vi "ApplyIconToLibrary.vi"(8 "error in (no error)":errorcluster, 9 "Apply banner color to class wire":bool=TRUE, 10 "Icon":refnum<class "Icon.lvclass">, 11 "Library Refnum in":refnum<vi>) -> (0 "error out":errorcluster, 3 "Library Refnum out":refnum<vi>)   [LabVIEW 2014, in "BasicClassDocumentation.lvlib" / "BasicClassDocumentation.lvclass"]
uses:
  BasicClassDocumentation.lvclass
  <vilib>/LabVIEW Icon API/lv_icon/Classes/Icon/Icon.lvclass
  <vilib>/LabVIEW Icon API/LabVIEW Icon API.lvlib
  Utilites/_ProjectItemsUtilities/_ProjectItemsUtilities.lvlib
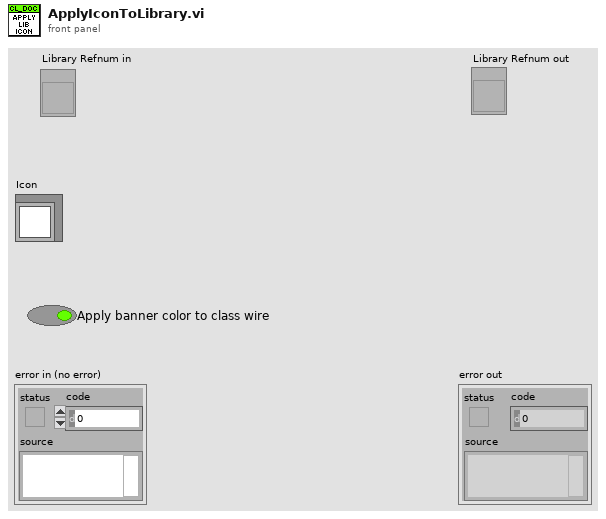
[diagram p1: front panel]
types:
  T1 = typedef "imagedata.ctl" = cluster{"image type":i32, "image depth":i32, "image":u8[], "mask":u8[], "colors":u32[], "Rectangle":cluster{"left":i16, "top":i16, "right":i16, "bottom":i16}}
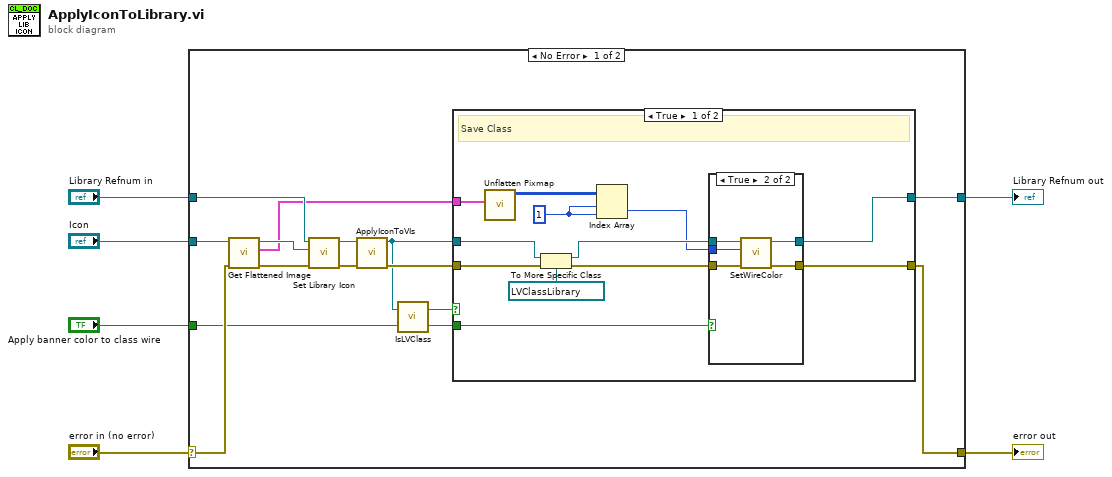
[diagram p0: block diagram]
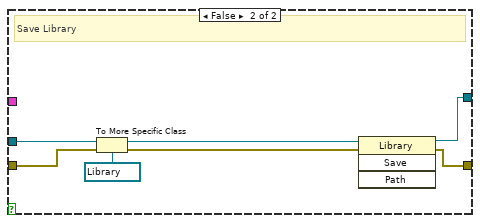
[diagram p3: hidden frame]
diagram:
  n1 = case shown="No Error" "error in (no error)" {
    selector: "error in (no error)" -> [w12 w48]
    tunnel: [w10 w48] -> w5
    tunnel: "Icon" -> [w14 _]
    tunnel: "Library Refnum in" -> [w15 w47]
    tunnel: [w8 w47] -> w2
    tunnel: "Apply banner color to class wire" -> [w7 _]
    frame No Error {
      n2 = call <vilib>:"Get Flattened Image.vi"("error in (no error)"=w12, "lv_icon.lvlib:Icon.lvclass in"=w14) -> ("error out"=w11:errorcluster, "Color Image"=w9:T1, "lv_icon.lvlib:Icon.lvclass out"=w13:refnum<class "Icon.lvclass">)  [unwired: 6 in, 1 out]
      n3 = call <vilib>:"Set Library Icon.vi"("error in (no error)"=w11, "Icon"=w13, "Library Refnum in"=w15) -> ("error out"=w20:errorcluster, "Library Refnum out"=w19:refnum<vi>)  [unwired: 7 in]
      n4 = call "ApplyIconToVIs.vi"("error in (no error)"=w20, "Library Refnum"=w19) -> ("error out"=w18:errorcluster, "Library Refnum out"=w17:refnum<vi>)  [unwired: 8 in]
      n5 = call "IsLVClass.vi"("ProjectItem Refnum"=w17) -> ("IsLVClass?"=w16:bool)  [unwired: 2 in]
      n6 = case shown="True" w16 {
        tunnel: w18 -> [w32 w46]
        tunnel: w17 -> [w29 w44]
        tunnel: w9 -> [w26 _]
        tunnel: [w31 w41] -> w10
        tunnel: [w22 w40] -> w8
        tunnel: w7 -> [w21 _]
        frame True {
          w24 = 1 ("index (row)")
          # "Save Class"
          n7 = call <vilib>:"Unflatten Pixmap.vi"("image data"=w26) -> ("24-bit pixmap"=w25:u32[][])  [unwired: 4 in, 6 out]
          n8 = To More Specific Class(target class=refnum<vi> refnum ("LVClassLibrary Refnum"), reference=w29, error in=w32) -> (specific class reference=w28:refnum<vi>, error out=w30:errorcluster)
          n9 = Index Array(array=w25, index (row)=w24, index (col)=w24) -> (element=w23:u32)
          n10 = case shown="True" w21 {
            tunnel: [w34 w39] -> w31
            tunnel: w30 -> [w34 w38]
            tunnel: w28 -> [w33 w37]
            tunnel: w23 -> [_ w36]
            tunnel: [w33 w35] -> w22
            frame False {
            }
            frame True {
              n11 = call "SetWireColor.vi"("error in (no error)"=w38, "Color"=w36, "LVClassLibrary Refnum"=w37) -> ("error out"=w39:errorcluster, "Library Refnum out"=w35:refnum<vi>)  [unwired: 7 in]
            }
          }
        }
        frame False {
          # "Save Library"
          n12 = To More Specific Class(target class=refnum<vi> refnum ("Library Refnum"), reference=w44, error in=w46) -> (specific class reference=w42:refnum<vi>, error out=w45:errorcluster)
          n13 = invoke class="Library" method="Save"(reference=w42, error in=w45) -> (reference out=w40:refnum<vi>, error out=w41:errorcluster)  [unwired: 2 in, 2 out]
        }
      }
    }
    frame Error {
    }
  }
  "error out" <- w5
  "Library Refnum out" <- w2
